vi "LitePoint_VSGConfig_CW_Waveform.vi"(8 "error in (no error)":errorcluster, 9 "WaveformBW":u16(ring) items=["20 MHz", "100 MHz"], 10 "Transmission":u16(ring) items=["CW", "Waveform"], 11 "VISA resource name":refnum<visa-resource-name>="LitePoint_IQxstream") -> (0 "error out":errorcluster, 3 "VISA resource name out":refnum<visa-resource-name>="LitePoint_IQxstream")   [LabVIEW 2020, in "LitePoints.lvlib"]
uses:
  LitePoints.lvlib
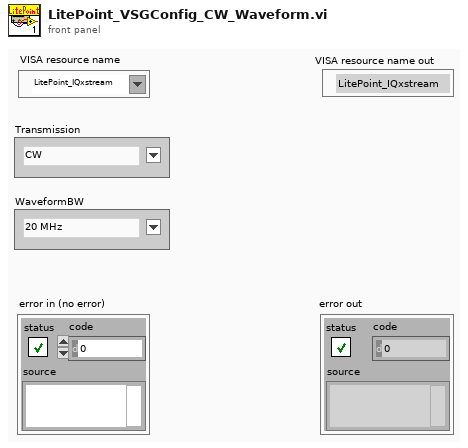
[diagram p1: front panel]
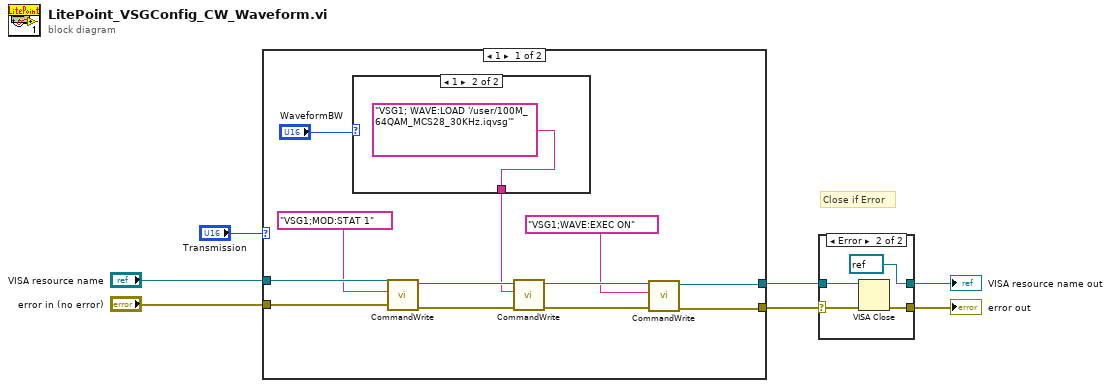
[diagram p0: block diagram]
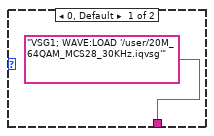
[diagram p2: hidden frame]
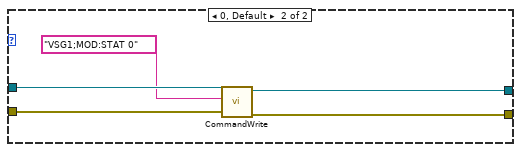
[diagram p3: hidden frame]
diagram:
  # "Close if Error"
  n1 = case shown="1" "Transmission" {
    tunnel: "VISA resource name" -> [w19 w26]
    tunnel: "error in (no error)" -> [w18 w25]
    tunnel: [w9 w24] -> w3
    tunnel: [w10 w23] -> w2
    frame 1 {
      n2 = case shown="1" "WaveformBW" {
        tunnel: ["VSG1; WAVE:LOAD '/user/20M_64QAM_MCS28_30KHz.iqvsg'" "VSG1; WAVE:LOAD '/user/100M_64QAM_MCS28_30KHz.iqvsg'"] -> w14
        frame 0, Default {
        }
        frame 1 {
        }
      }
      n3 = call "CommandWrite.vi"("error in (no error)"=w18, "Write Buffer"="VSG1;MOD:STAT 1", "VISA resource name"=w19) -> ("error out"=w16:errorcluster, "VISA resource name out"=w17:refnum<visa-resource-name>)  [unwired: 7 in]
      n4 = call "CommandWrite.vi"("error in (no error)"=w16, "Write Buffer"=w14, "VISA resource name"=w17) -> ("error out"=w11:errorcluster, "VISA resource name out"=w12:refnum<visa-resource-name>)  [unwired: 7 in]
      n5 = call "CommandWrite.vi"("error in (no error)"=w11, "Write Buffer"="VSG1;WAVE:EXEC ON", "VISA resource name"=w12) -> ("error out"=w10:errorcluster, "VISA resource name out"=w9:refnum<visa-resource-name>)  [unwired: 7 in]
    }
    frame 0, Default {
      n6 = call "CommandWrite.vi"("error in (no error)"=w25, "Write Buffer"="VSG1;MOD:STAT 0", "VISA resource name"=w26) -> ("error out"=w23:errorcluster, "VISA resource name out"=w24:refnum<visa-resource-name>)  [unwired: 7 in]
    }
  }
  n7 = case shown="Error" w2 {
    selector: w2 -> [w27 w30]
    tunnel: w3 -> [w28 w31]
    tunnel: [w28 refnum<visa-resource-name> refnum ("VISA resource name out")] -> w7
    tunnel: [w27 w29] -> w6
    frame No Error {
    }
    frame Error {
      n8 = VISA Close(VISA resource name=w31, error in (no error)=w30) -> (error out=w29:errorcluster)
    }
  }
  "VISA resource name out" <- w7
  "error out" <- w6
